vi "manager.vi"(8 "error in (no error)":errorcluster, 9 "control references":T1, 10 "top-level VI ref in":refnum<vi>, 11 "GenericToplevelComponent in":refnum<class "GenericToplevelComponent.lvclass">) -> (0 "error out":errorcluster, 2 "top-level VI ref out":refnum<vi>, 3 "GenericToplevelComponent out":refnum<class "GenericToplevelComponent.lvclass">)   [LabVIEW 2010, in "GenericToplevelComponent.lvclass"]
uses:
  GenericToplevelComponent.lvclass
  main/labview_source/type_definitions/clusters/controls_refs.ctl
  ErrorController/ErrorController/class_data.vi
  ErrorController/ErrorController/ErrorController.lvclass
panel:
  out "loop counter":i32
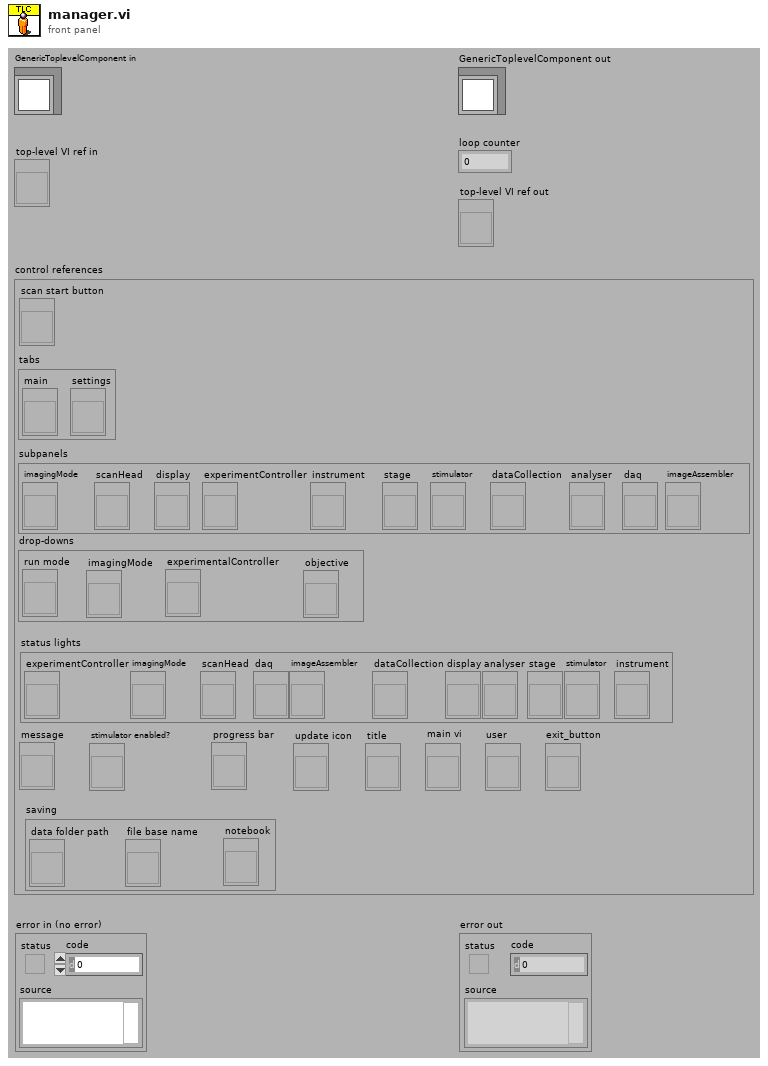
[diagram p1: front panel]
types:
  T1 = typedef "controls_refs.ctl" = cluster{"scan start button":refnum<vi>, "tabs":cluster{"main":refnum<vi>, "settings":refnum<vi>}, "subpanels":cluster{"imagingMode":refnum<vi>, "scanHead":refnum<vi>, "display":refnum<vi>, "experimentController":refnum<vi>, "instrument":refnum<vi>, "stage":refnum<vi>, "stimulator":refnum<vi>, "dataCollection":refnum<vi>, "analyser":refnum<vi>, "daq":refnum<vi>, "imageAssembler":refnum<vi>}, "drop-downs":cluster{"run mode":refnum<vi>, "imagingMode":refnum<vi>, "experimentalController":refnum<vi>, "objective":refnum<vi>}, "status lights":cluster{"experimentController":refnum<vi>, "imagingMode":refnum<vi>, "scanHead":refnum<vi>, "daq":refnum<vi>, "imageAssembler":refnum<vi>, "dataCollection":refnum<vi>, "display":refnum<vi>, "analyser":refnum<vi>, "stage":refnum<vi>, "stimulator":refnum<vi>, "instrument":refnum<vi>}, "message":refnum<vi>, "stimulator enabled?":refnum<vi>, "saving":cluster{"data folder path":refnum<vi>, "file base name":refnum<vi>, "notebook":refnum<vi>}, "progress bar":refnum<vi>, "update icon":refnum<vi>, "title":refnum<vi>, "main vi":refnum<vi>, "user":refnum<vi>, "exit_button":refnum<vi>}
  T2 = typedef "main_trigger_enum.ctl" = enum16{"NULL", "initialise", "terminate", "start", "stop", "change objective", "change experimentController", "change imagingMode", "save notebook", "started saving", "finished saving", "expCtr ready", "expCtr missing", "imgMd ready", "imgMd missing", "scanHd ready", "scanHd missing", "DAQ ready", "DAQ missing", "imgAsm ready", "imgAsm missing", "dataColl ready", "dataColl missing", "display ready", "display missing", "analysr ready", "analysr missing", "instrmnt ready", "instrmnt missing", "stimltr ready", "stimltr missing", "stage ready", "stage missing"}
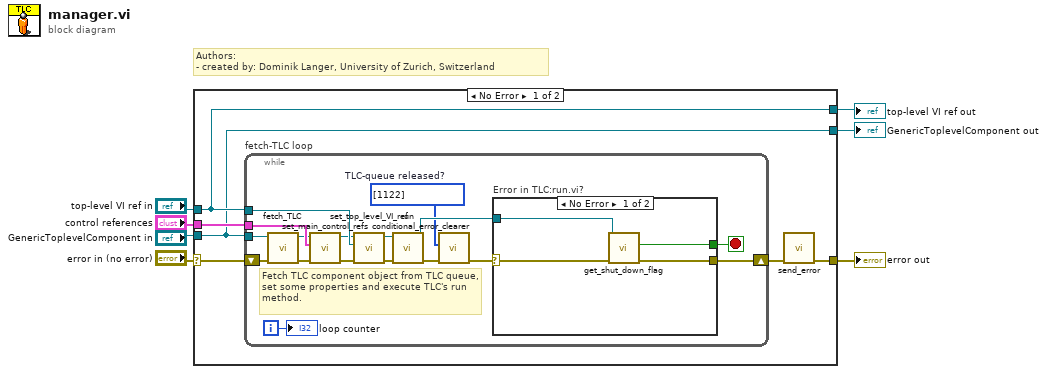
[diagram p0: block diagram]
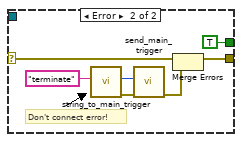
[diagram p2: hidden frame]
diagram:
  # "Authors: \n- created by: Dominik Langer, University of Zurich, Switzerland"
  n1 = case shown="No Error" "error in (no error)" {
    selector: "error in (no error)" -> [w13 w44]
    tunnel: [w8 w44] -> w3
    tunnel: "control references" -> [w12 _]
    tunnel: "top-level VI ref in" -> [w11 w43]
    tunnel: [w11 w43] -> w5
    tunnel: "GenericToplevelComponent in" -> [w9 w42]
    tunnel: [w9 w42] -> w1
    frame No Error {
      n2 = while "fetch-TLC loop" {
        tunnel: w12 -> [w30]
        tunnel: w11 -> [w26]
        tunnel: w9 -> [w17]
        shift-right: [w19] -> w10
        shift-left: w13 -> [w29]
        i -> [w16]
        stop <- w14 stop-if-true
        w22 = i32[] [1122]  # TLC-queue released?
        # "Fetch TLC component object from TLC queue, set some properties and execute TLC's run method."
        n3 = call-dynamic "fetch_TLC.vi"("error in (no error)"=w29, "GenericToplevelComponent in"=w17) -> ("error out"=w28:errorcluster, "GenericToplevelComponent out"=w18:refnum<class "GenericToplevelComponent.lvclass">)  [unwired: 8 in]
        n4 = call-dynamic "set_main_control_refs.vi"("error in (no error)"=w28, "control references"=w30, "GenericPlugin.lvclass in"=w18) -> ("error out"=w27:errorcluster, "GenericPlugin.lvclass out"=w25:refnum<class "GenericToplevelComponent.lvclass">)  [unwired: 7 out]
        n5 = call-dynamic "set_top_level_VI_ref.vi"("error in (no error)"=w27, "top-level VI ref"=w26, "GenericPlugin.lvclass in"=w25) -> ("error out"=w21:errorcluster, "GenericPlugin.lvclass out"=w20:refnum<class "GenericToplevelComponent.lvclass">)  [unwired: 7 out]
        n6 = call-dynamic "run.vi"("error in (no error)"=w21, "GenericToplevelComponent in"=w20) -> ("error out"=w23:errorcluster, "GenericToplevelComponent out"=w24:refnum<class "GenericToplevelComponent.lvclass">)  [unwired: 8 out]
        n7 = call "conditional_error_clearer.vi"("error in (no error)"=w23, "array of clearable error codes"=w22) -> ("error out"=w15:errorcluster)  [unwired: 1 in, 8 out]
        n8 = case "Error in TLC:run.vi?" shown="No Error" w15 {
          selector: w15 -> [w31 w37]
          tunnel: w24 -> [w34 _]
          tunnel: [w33 w35] -> w19
          tunnel: [w32 TRUE] -> w14
          frame No Error {
            n9 = call-dynamic "get_shut_down_flag.vi"("error in (no error)"=w31, "GenericPlugin in"=w34) -> ("error out"=w33:errorcluster, "shut down?"=w32:bool)  [unwired: 8 out]
          }
          frame Error {
            # "Don't connect error!"
            n10 = call "string_to_main_trigger.vi"("trigger string"="terminate") -> ("error out"=w40:errorcluster, "main trigger"=w39:T2)  [unwired: 9 in]
            n11 = call "send_main_trigger.vi"("error in (no error)"=w40, "trigger"=w39) -> ("error out"=w36:errorcluster)  [unwired: 9 in]
            n12 = Merge Errors(w37, w36) -> (w35:errorcluster)
          }
        }
        "loop counter" <- w16
      }
      n13 = call "send_error.vi"("error in (no error)"=w10) -> ("error out"=w8:errorcluster)  [unwired: 10 in]
    }
    frame Error {
    }
  }
  "error out" <- w3
  "GenericToplevelComponent out" <- w1
  "top-level VI ref out" <- w5
